vi "8.2.vi"() -> ()   [LabVIEW 2017]
panel:
  out "Numeric 2":u64
  out "Numeric":u64
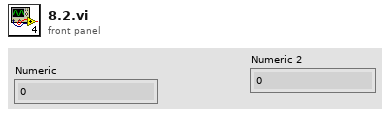
[diagram p1: front panel]
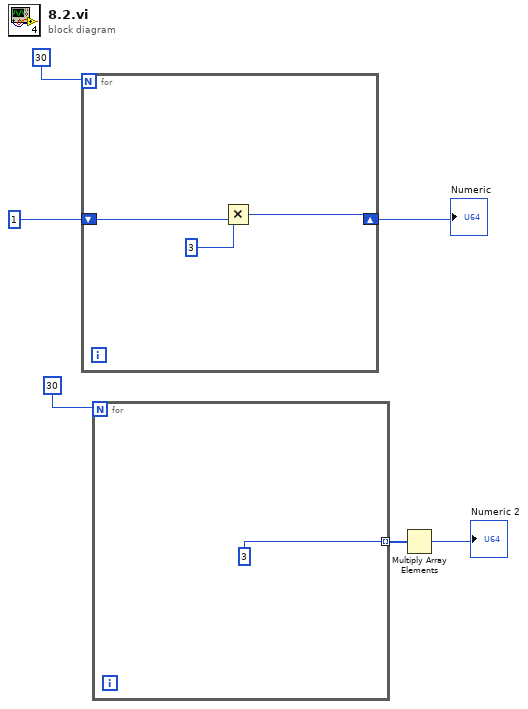
[diagram p0: block diagram]
diagram:
  n1 = for {
    N: 30 -> [_]
    shift-right: [w7] -> w4
    shift-left: 1 -> [w9]
    n2 = Multiply(x=w9, y=3) -> (x*y=w7:i32)
  }
  "Numeric" <- w4
  n3 = for {
    N: 30 -> [_]
    tunnel: [3] -> w2 mode=indexing
  }
  n4 = Multiply Array Elements(1:w2) -> (0:→"Numeric 2":i32)
